vi "test CE14(APIs).vi"() -> ()   [LabVIEW 2018]
uses:
  CE14_eMIC.lvlib
panel:
  in  "PF":bool
  in  "current":bool
  out "read buffer":string
  in  "voltage":bool
  in  "stop":bool
  out "Response msg":string[](array[string])
  in  "VISA resource name":refnum<visa-resource-name>="COM12"
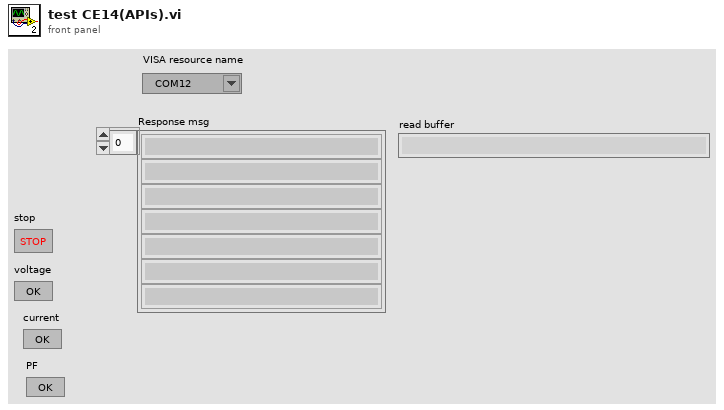
[diagram p1: front panel]
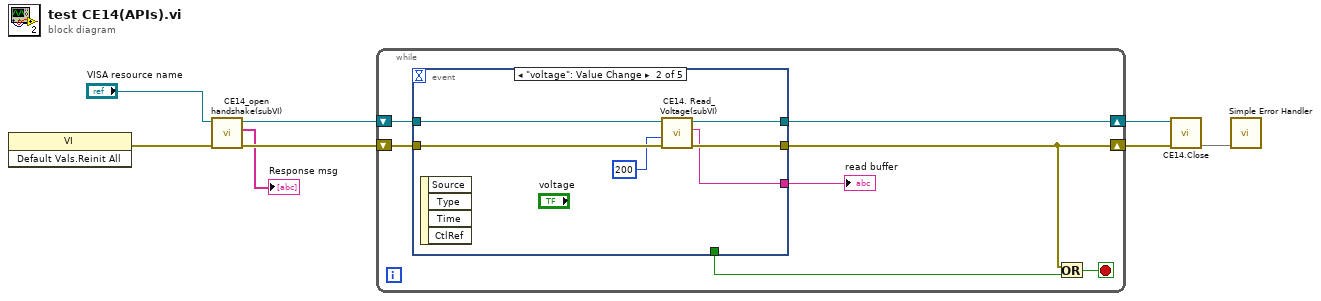
[diagram p0: block diagram]
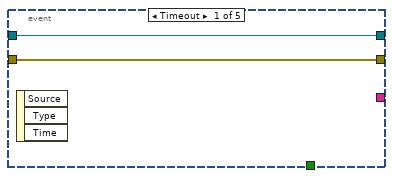
[diagram p2: hidden frame]
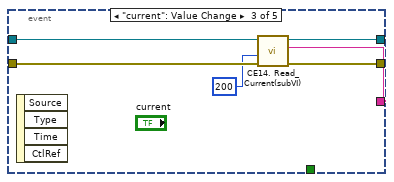
[diagram p3: hidden frame]
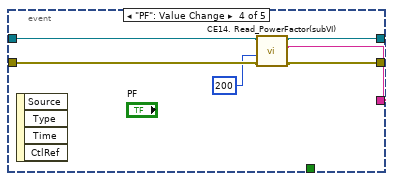
[diagram p4: hidden frame]
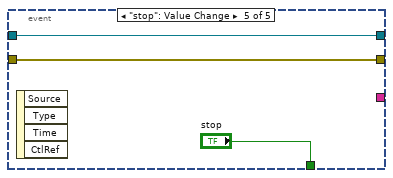
[diagram p5: hidden frame]
diagram:
  n1 = invoke class="VI" method="Default Vals.Reinit All"() -> (error out=w6:errorcluster)  [unwired: 3 in, 2 out]
  n2 = call "CE14_open handshake(subVI).vi"("error in(no error)"=w6, "VISA resource name"="VISA resource name") -> ("error out"=w5:errorcluster, "response msg"=→"Response msg":string[], "VISA resource name 2"=w7:refnum<visa-resource-name>)  [unwired: 6 in, 1 out]
  n3 = while {
    shift-right: [w13] -> w4
    shift-left: w7 -> [w15]
    shift-right: [w12] -> w3
    shift-left: w5 -> [w14]
    stop <- w10 stop-if-true
    n4 = event shown="[1] \"voltage\": Value Change" {
      selector: _ -> [_ _ _ _ _]
      dyn-events: _ -> [_ _ _ _ _]
      timeout: _ -> [_ _ _ _ _]
      tunnel: w15 -> [w17 w23 w29 w35 w38]
      tunnel: w14 -> [w16 w22 w28 w34 w37]
      tunnel: [w17 w21 w27 w32 w38] -> w13
      tunnel: [w16 w20 w26 w30 w37] -> w12
      tunnel: [_ _ _ _ "stop"] -> w11
      tunnel: [_ w19 w25 w31 _] -> w9
      event Timeout {
        n5 = event-data() -> ()  [unwired: 1 in, 3 out]
      }
      event "voltage": Value Change {
        n6 = event-data() -> ()  [unwired: 1 in, 4 out]
        n7 = call "CE14. Read_Voltage(subVI).vi"("error in (no error)"=w22, "milliseconds to wait(100)"=u32 200, "VISA resource name"=w23) -> ("error out"=w20:errorcluster, "read buffer"=w19:string, "VISA resource name out"=w21:refnum<visa-resource-name>)  [unwired: 5 in, 1 out]
      }
      event "current": Value Change {
        n8 = event-data() -> ()  [unwired: 1 in, 4 out]
        n9 = call "CE14. Read_Current(subVI).vi"("error in (no error)"=w28, "milliseconds to wait(200)"=u32 200 ("milliseconds to wait(100)"), "VISA resource name"=w29) -> ("error out"=w26:errorcluster, "received msg"=w25:string, "VISA resource name out"=w27:refnum<visa-resource-name>)  [unwired: 5 in, 1 out]
      }
      event "PF": Value Change {
        n10 = event-data() -> ()  [unwired: 1 in, 4 out]
        n11 = call "CE14. Read_PowerFactor(subVI).vi"("error in (no error)"=w34, "milliseconds to wait(200)"=u32 200 ("milliseconds to wait(100)"), "VISA resource name"=w35) -> ("error out"=w30:errorcluster, "read buffer"=w31:string, "VISA resource name out"=w32:refnum<visa-resource-name>)  [unwired: 5 in, 1 out]
      }
      event "stop": Value Change {
        n12 = event-data() -> ()  [unwired: 1 in, 4 out]
      }
    }
    "read buffer" <- w9
    n13 = Or(x=w12, y=w11) -> (x .or. y?=w10:bool)
  }
  n14 = call "CE14.Close.vi"(8:w3, 11:w4) -> (0:w2)  [unwired: 9 in]
  n15 = call <vilib>:"Simple Error Handler.vi"("error in (no error)"=w2) -> ()  [unwired: 4 in, 5 out]
